vi "2exp fit cs.vi"(0 "S+B":dbl format="%.2f", 1 "biExp fit":bool, 2 "B":dbl=500.0 format="%.2f", 3 "y":dbl[](array[numeric]), 4 "Autocorr data":cluster{dbl[], "Best Fit":dbl[]}[](graph), 5 "x":dbl[](array[numeric])) -> (6 "best fit":dbl[](array[numeric]) caption="best fit output", 7 "results":cluster{dbl, dbl, dbl, dbl, dbl, dbl}, 8 "x-values":dbl[](array[numeric]))   [LabVIEW 2009]
uses:
  Instance           4 19Saved   2exp fit cs .vi
  Instance           5 19Saved   2exp fit cs .vi
  Instance           3 19Saved   2exp fit cs .vi
  Instance           2 19Saved   2exp fit cs .vi
  Instance           6 19Saved   2exp fit cs .vi
  Instance           1 19Saved   2exp fit cs .vi
panel:
  out "t_off 2":dbl
  out "t_on 2":dbl
  out "A2 corrected":dbl
  out "t_on1":dbl
  out "t_off 1":dbl
  out "A1 corrected":dbl format="%.2f"
  out "t2":dbl
  out "t1":dbl
  out "A2":dbl
  out "A1":dbl
  out "best fit":dynamicdata(graph) caption="Beste Anpassung"
  # "Inputs"
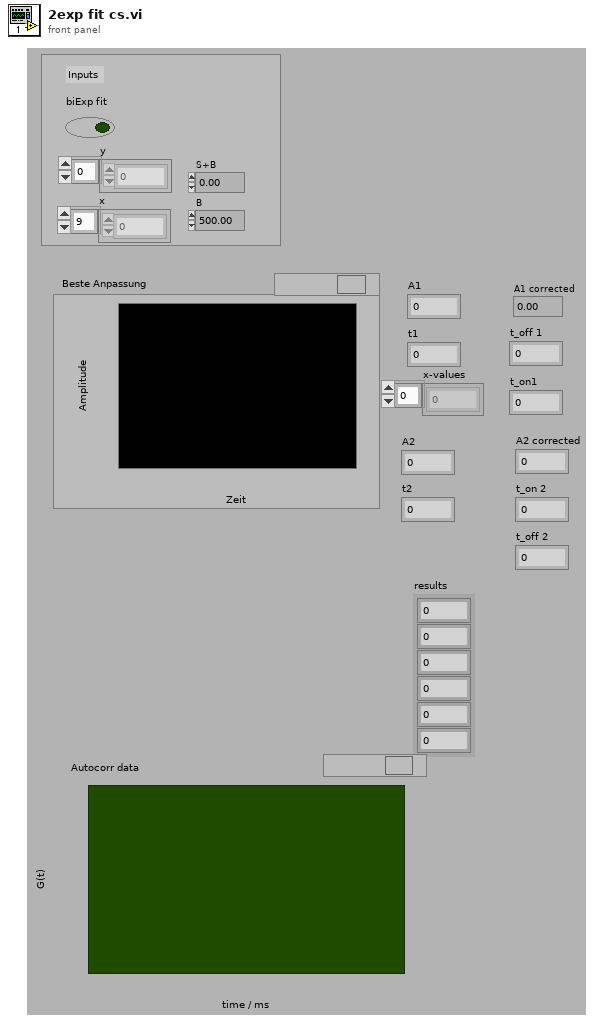
[diagram p1: front panel]
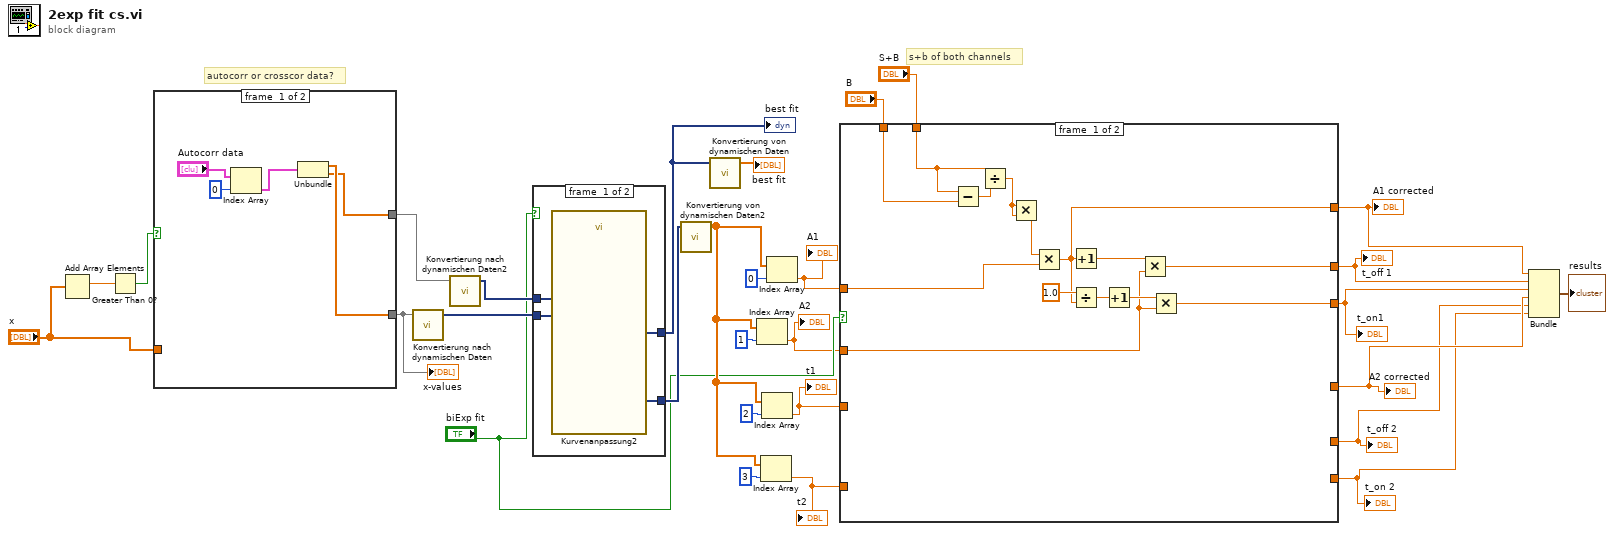
[diagram p0: block diagram]
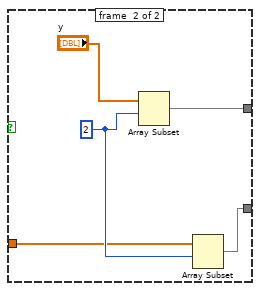
[diagram p2: hidden frame]
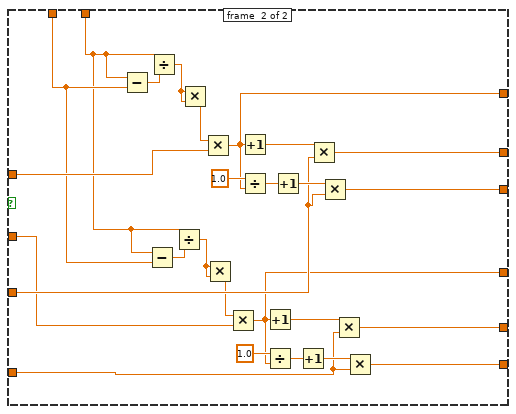
[diagram p3: hidden frame]
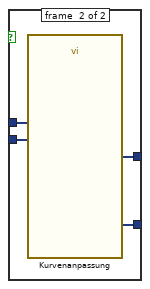
[diagram p4: hidden frame]
diagram:
  # "s+b of both channels"
  # "autocorr or crosscor data?"
  n1 = Add Array Elements(numeric array="x") -> (sum=w2:dbl)
  n2 = Greater Than 0?(x=w2) -> (x > 0?=w1:bool)
  n3 = case shown="False" w1 {
    tunnel: [w30 w38] -> w21
    tunnel: [w31 w36] -> w20
    tunnel: "x" -> [_ w35]
    frame #0 {
      n4 = Index Array(array="Autocorr data", index=0) -> (element=w32:cluster{dbl[], "Best Fit":dbl[]})
      n5 = Unbundle(w32) -> (w31:dbl[], "Best Fit"=w30:dbl[])
    }
    frame #1 {
      w39 = 2 ("Index")
      n6 = Array Subset(array="y", index=w39) -> (w38:dbl[])  [unwired: 1 in]
      n7 = Array Subset(array=w35, index=w39) -> (w36:dbl[])  [unwired: 1 in]
    }
  }
  "x-values" <- w20
  n8 = call "Konvertierung nach dynamischen Daten"("Array"=w20) -> ("Dynamic Data Type"=w18:dynamicdata)  [unwired: 3 in]
  n9 = call "Konvertierung nach dynamischen Daten2"("Array"=w21) -> ("Dynamic Data Type"=w19:dynamicdata)  [unwired: 3 in]
  n10 = case shown="True" "biExp fit" {
    tunnel: [w43 w47] -> w23
    tunnel: [w42 w46] -> w22
    tunnel: w19 -> [w41 w45]
    tunnel: w18 -> [w40 w44]
    frame #0 {
      n11 = call "Kurvenanpassung2"("Locations"=w40, "Signals"=w41) -> ("best fit"=w43:dynamicdata, "non-linear coefficients"=w42:dynamicdata)  [unwired: 5 in, 3 out]
    }
    frame #1 {
      n12 = call "Kurvenanpassung"("Locations"=w44, "Signals"=w45) -> ("best fit"=w47:dynamicdata, "non-linear coefficients"=w46:dynamicdata)  [unwired: 5 in, 3 out]
    }
  }
  "best fit" <- w23
  n13 = call "Konvertierung von dynamischen Daten2"("Dynamic Data Type"=w22) -> ("Array"=w29:dbl[])  [unwired: 3 in]
  n14 = call "Konvertierung von dynamischen Daten"("Dynamic Data Type"=w23) -> ("Array"=→"best fit":dbl[])  [unwired: 3 in]
  n15 = Index Array(array=w29, index=1 ("Index")) -> (element=w12:dbl)
  "A2" <- w12
  n16 = Index Array(array=w29, index=3 ("Index")) -> (element=w11:dbl)
  "t2" <- w11
  n17 = Index Array(array=w29, index=2 ("Index")) -> (element=w15:dbl)
  "t1" <- w15
  n18 = Index Array(array=w29, index=0 ("Index")) -> (element=w16:dbl)
  "A1" <- w16
  n19 = case shown="False" "biExp fit" {
    tunnel: w16 -> [w58 w84]
    tunnel: w15 -> [_ w79]
    tunnel: [w53 w78] -> w10
    tunnel: [w52 w77] -> w9
    tunnel: [w51 w76] -> w8
    tunnel: "S+B" -> [w50 w67]
    tunnel: "B" -> [w49 w68]
    tunnel: w12 -> [w48 w66]
    tunnel: [_ w65] -> w7
    tunnel: w11 -> [_ w64]
    tunnel: [_ w63] -> w5
    tunnel: [_ w62] -> w6
    frame #0 {
      n20 = Subtract(x=w50, y=w49) -> (x-y=w61:dbl)
      n21 = Divide(x=w50, y=w61) -> (x/y=w60:dbl)
      n22 = Multiply(x=w60, y=w60) -> (x*y=w59:dbl)
      n23 = Multiply(x=w59, y=w58) -> (x*y=w53:dbl)
      n24 = Increment(x=w53) -> (x+1=w57:dbl)
      n25 = Divide(x=1.0, y=w53) -> (x/y=w55:dbl)
      n26 = Increment(x=w55) -> (x+1=w54:dbl)
      n27 = Multiply(x=w57, y=w48) -> (x*y=w52:dbl)
      n28 = Multiply(x=w54, y=w48) -> (x*y=w51:dbl)
    }
    frame #1 {
      n29 = Subtract(x=w67, y=w68) -> (x-y=w87:dbl)
      n30 = Subtract(x=w67, y=w68) -> (x-y=w75:dbl)
      n31 = Divide(x=w67, y=w87) -> (x/y=w86:dbl)
      n32 = Divide(x=w67, y=w75) -> (x/y=w74:dbl)
      n33 = Multiply(x=w86, y=w86) -> (x*y=w85:dbl)
      n34 = Multiply(x=w85, y=w84) -> (x*y=w78:dbl)
      n35 = Multiply(x=w74, y=w74) -> (x*y=w73:dbl)
      n36 = Multiply(x=w73, y=w66) -> (x*y=w65:dbl)
      n37 = Increment(x=w78) -> (x+1=w83:dbl)
      n38 = Divide(x=1.0, y=w78) -> (x/y=w81:dbl)
      n39 = Increment(x=w65) -> (x+1=w72:dbl)
      n40 = Divide(x=1.0, y=w65) -> (x/y=w70:dbl)
      n41 = Increment(x=w81) -> (x+1=w80:dbl)
      n42 = Increment(x=w70) -> (x+1=w69:dbl)
      n43 = Multiply(x=w83, y=w79) -> (x*y=w77:dbl)
      n44 = Multiply(x=w80, y=w79) -> (x*y=w76:dbl)
      n45 = Multiply(x=w72, y=w64) -> (x*y=w62:dbl)
      n46 = Multiply(x=w69, y=w64) -> (x*y=w63:dbl)
    }
  }
  "t_off 1" <- w9
  "t_on1" <- w8
  "A1 corrected" <- w10
  "A2 corrected" <- w7
  "t_on 2" <- w5
  "t_off 2" <- w6
  n47 = Bundle(w10, w9, w8, w7, w6, w5) -> (→"results":cluster{dbl, dbl, dbl, dbl, dbl, dbl})  [unwired: 1 in]
